vi "Comm String Send CMD.vi"(0 "niDTS Comm Telnet in":refnum<class "niDTS Comm Telnet.lvclass">, 5 "Command":string, 11 "error in (no error)":errorcluster) -> (4 "niDTS Comm Telnet out":refnum<class "niDTS Comm Telnet.lvclass">, 15 "error out":errorcluster)   [LabVIEW 2015, in "niDTS CommLib.lvlib" / "niDTS Comm Telnet.lvclass"]
doc: "Send the raw command over the Telnet port. This does NOT prepend the cmdPrefix to the command. For that functionality, use Comm String Send Command."
uses:
  niDTS Comm Telnet.lvclass
  niDTS Comm Telnet.lvclass/niDTS Comm Telnet.ctl
  Utility/telnet/NI_InternetTK_Core_VIs.lvlib
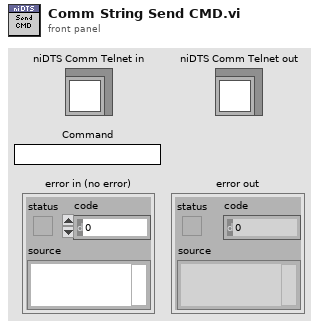
[diagram p1: front panel]
types:
  T1 = typedef "Telnet Session.ctl" = refnum<k1>
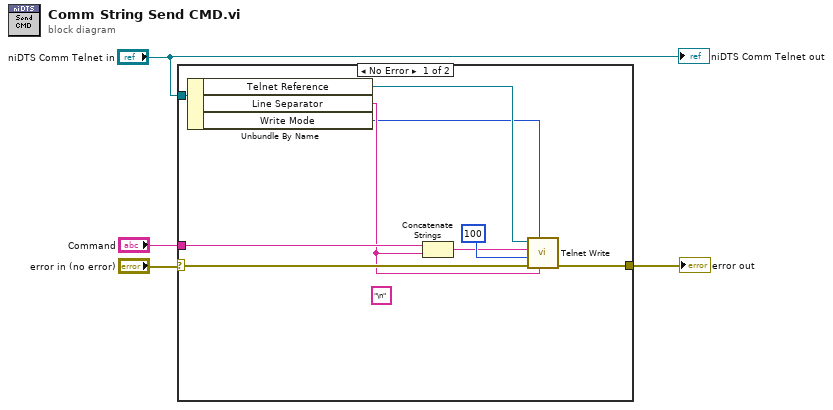
[diagram p0: block diagram]
diagram:
  n1 = case shown="No Error" "error in (no error)" {
    selector: "error in (no error)" -> [w7 w14]
    tunnel: "niDTS Comm Telnet in" -> [w10 _]
    tunnel: "Command" -> [w9 _]
    tunnel: [w8 w14] -> w3
    frame No Error {
      (unwired) "\n" ("string")
      n2 = Unbundle By Name(w10) -> ("Telnet Reference"=w11:T1, "Line Separator"=w6:string, "Write Mode"=w5:enum16{"normal", "line", "buffered"})
      n3 = Concatenate Strings(w9, w6) -> (w12:string)
      n4 = call "Telnet Write.vi"("line separator (\\n)"=w6, "write mode (normal)"=w5, "error in (no error)"=w7, "timeout ms (25000)"=100, "data in"=w12, "telnet connection"=w11) -> ("error out"=w8:errorcluster)  [unwired: 1 in, 2 out]
    }
    frame Error {
    }
  }
  "error out" <- w3
  "niDTS Comm Telnet out" <- "niDTS Comm Telnet in"
